vi "pulses to angle.vi"(11 "Pulses":dbl) -> (3 "Angle":dbl)   [LabVIEW 2025, in "Motor.lvlib" / "CL57RS.lvclass"]
uses:
  CL57RS.lvclass
  CL57RS.lvclass/CL57RS.ctl
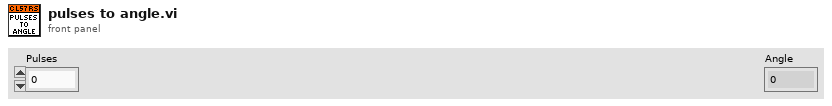
[diagram p1: front panel]
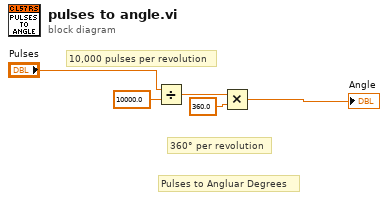
[diagram p0: block diagram]
diagram:
  # "Pulses to Angluar Degrees"
  # "360° per revolution"
  # "10,000 pulses per revolution"
  n1 = Divide(x="Pulses", y=10000.0) -> (x/y=w5:dbl)
  n2 = Multiply(x=w5, y=360.0) -> (x*y=→"Angle":dbl)
